vi "LabVIEW2.vi"() -> ()   [LabVIEW 2023]
uses:
  <vilib>/Utility/error.llb/Trim Whitespace One-Sided.vi
panel:
  in  "PNG file path":path=path "/Users/leogallacio/Downloads/N8.png"
  out "concatenated string":string
  out "name":string
  out "Extract path":path
  out "spreadsheet string 2":string
  out "Array 2":string[](array[string])
  out "spreadsheet string":string
  in  "Marker size":i32
  in  "Marker shape":string
  out "Array":u8[][](array[numeric])
  out "appended array":u8[](array[numeric])
  out "B":u8
  out "G":u8
  out "R":u8
  out "size(s)":i32
  out "array":i32[](array[numeric])
  out "before substring":string
  out "after substring":string
  out "Corners":u32(colorbox)
  out "Traces":u32[](array[colorbox])
  out "Color Box":u32(colorbox)
  out "Array with the 6 colors of stdout":i32[](array[numeric])
  out "C:":string
  out "Corners":i32
  out "Color CLUT at index I":u32
  out "CLUT":u32[](array[numeric])
  out "standard error 2":string
  out "standard output 2":string
  out "error out 2":errorcluster
  out "resulting string":string
  out "script.m path":path
  out "return path":path
  out "Traces.txt path":path
  out "name :\nLabVIEW1.vi":string
  out "Traces.txt":string
  out "error out":errorcluster
  out "standard error":string
  out "standard output":string
  out "LabBIEW path :\n/Users/leogallacio/Downloads/LabVIEW":path
  out "Pixmap.bin path":path
  out "profondeur":i32
  out "image":u8[](array[numeric])
  out "largeur":i16
  out "hauteur":i16
  out "PNG picture":picture
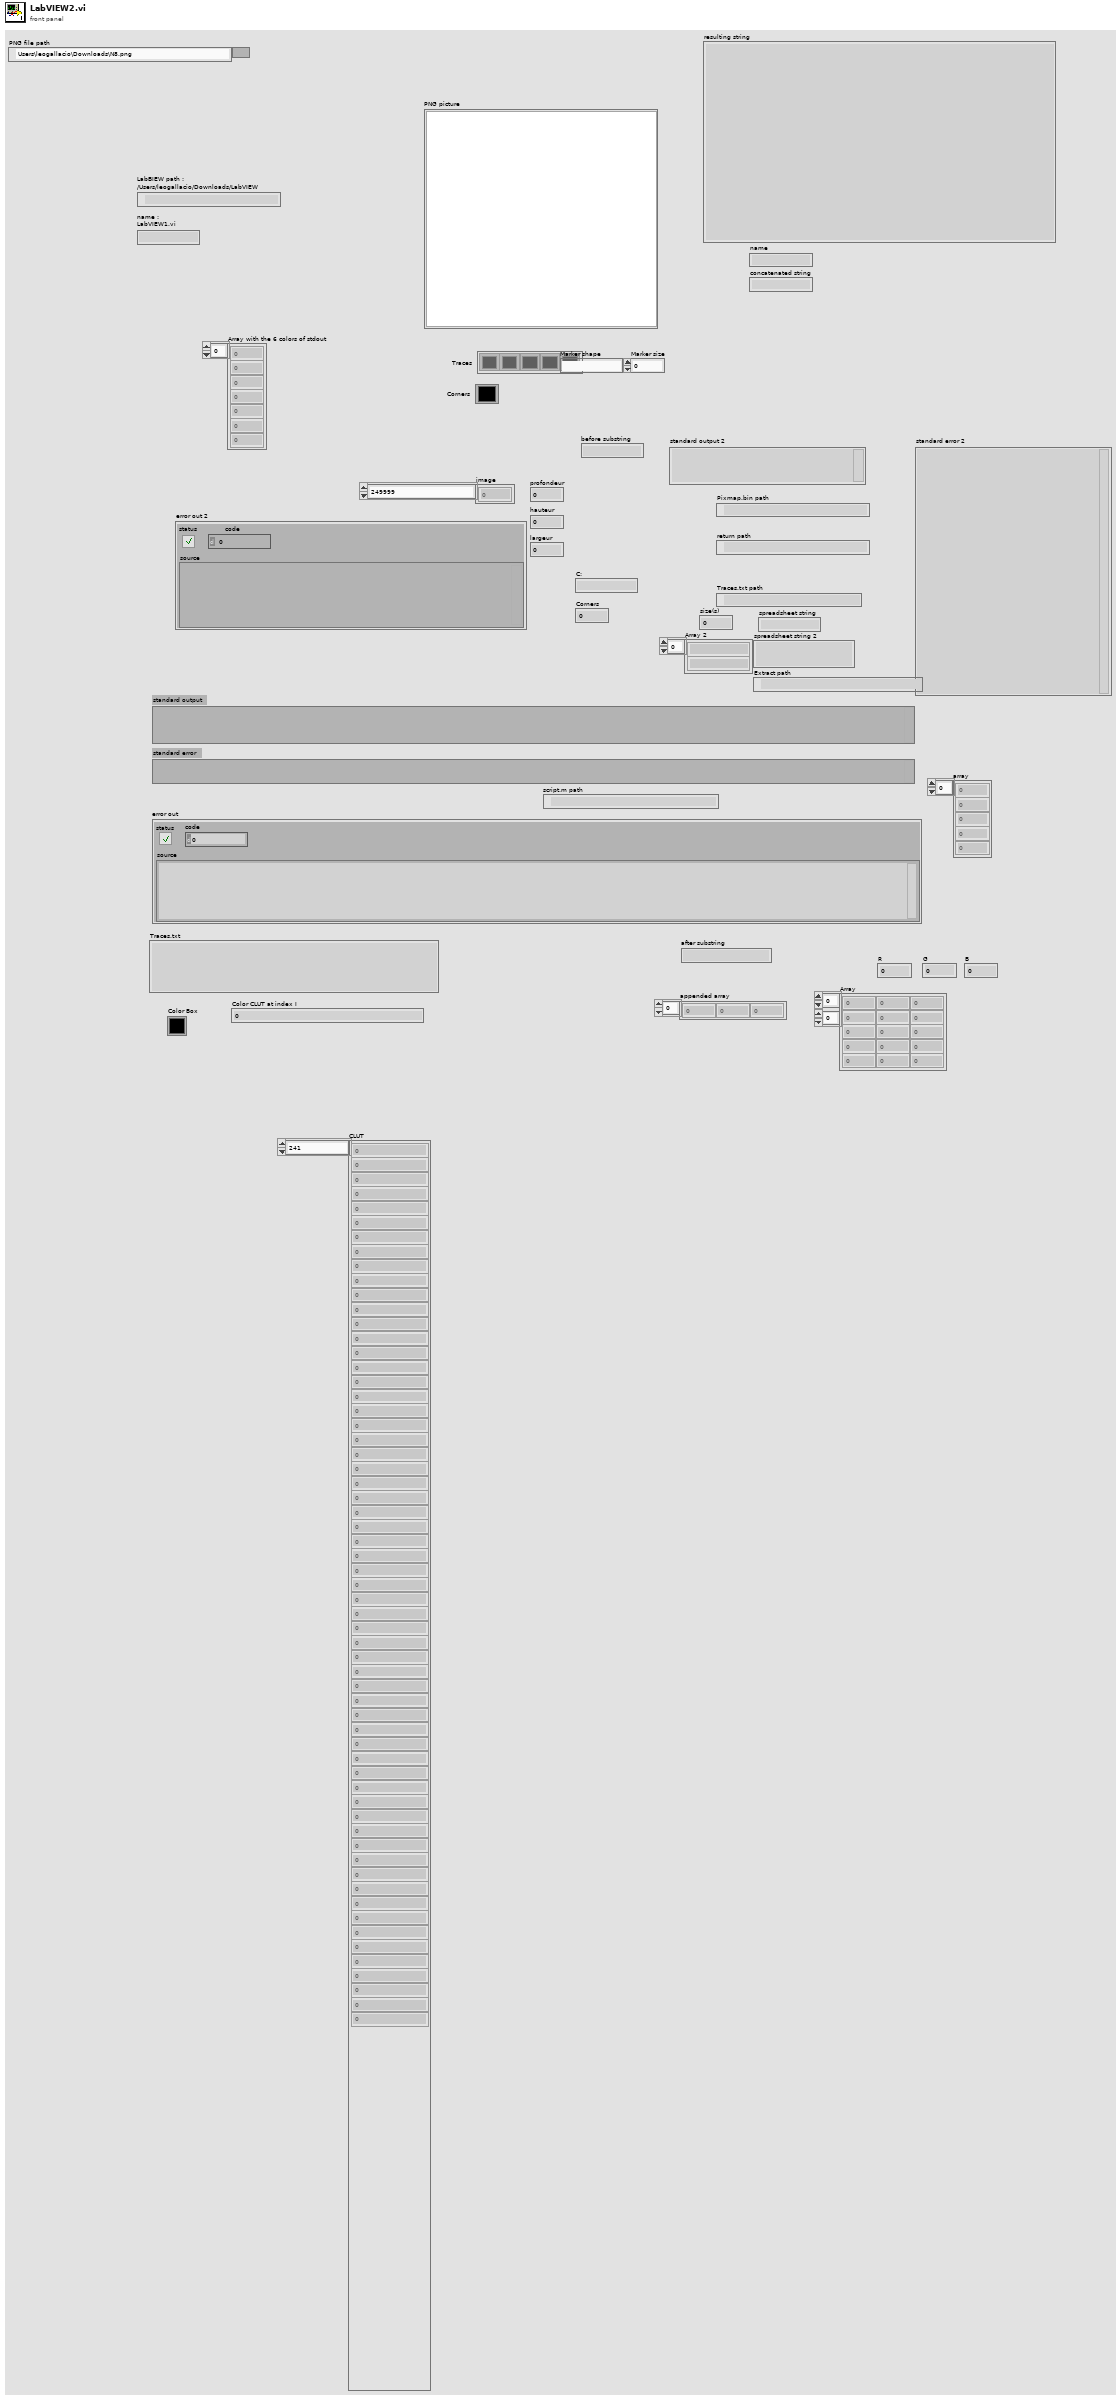
[diagram p1: front panel]
types:
  T1 = enum16{"open", "replace", "create", "open or create", "replace or create", "replace or create with confirmation"}
  T2 = enum16{"big-endian, network order", "native, host order", "little-endian"}
  T3 = typedef "imagedata.ctl" = cluster{"image type":i32, "image depth":i32, "image":u8[], "mask":u8[], "colors":u32[], "Rectangle":cluster{"left":i16, "top":i16, "right":i16, "bottom":i16}}
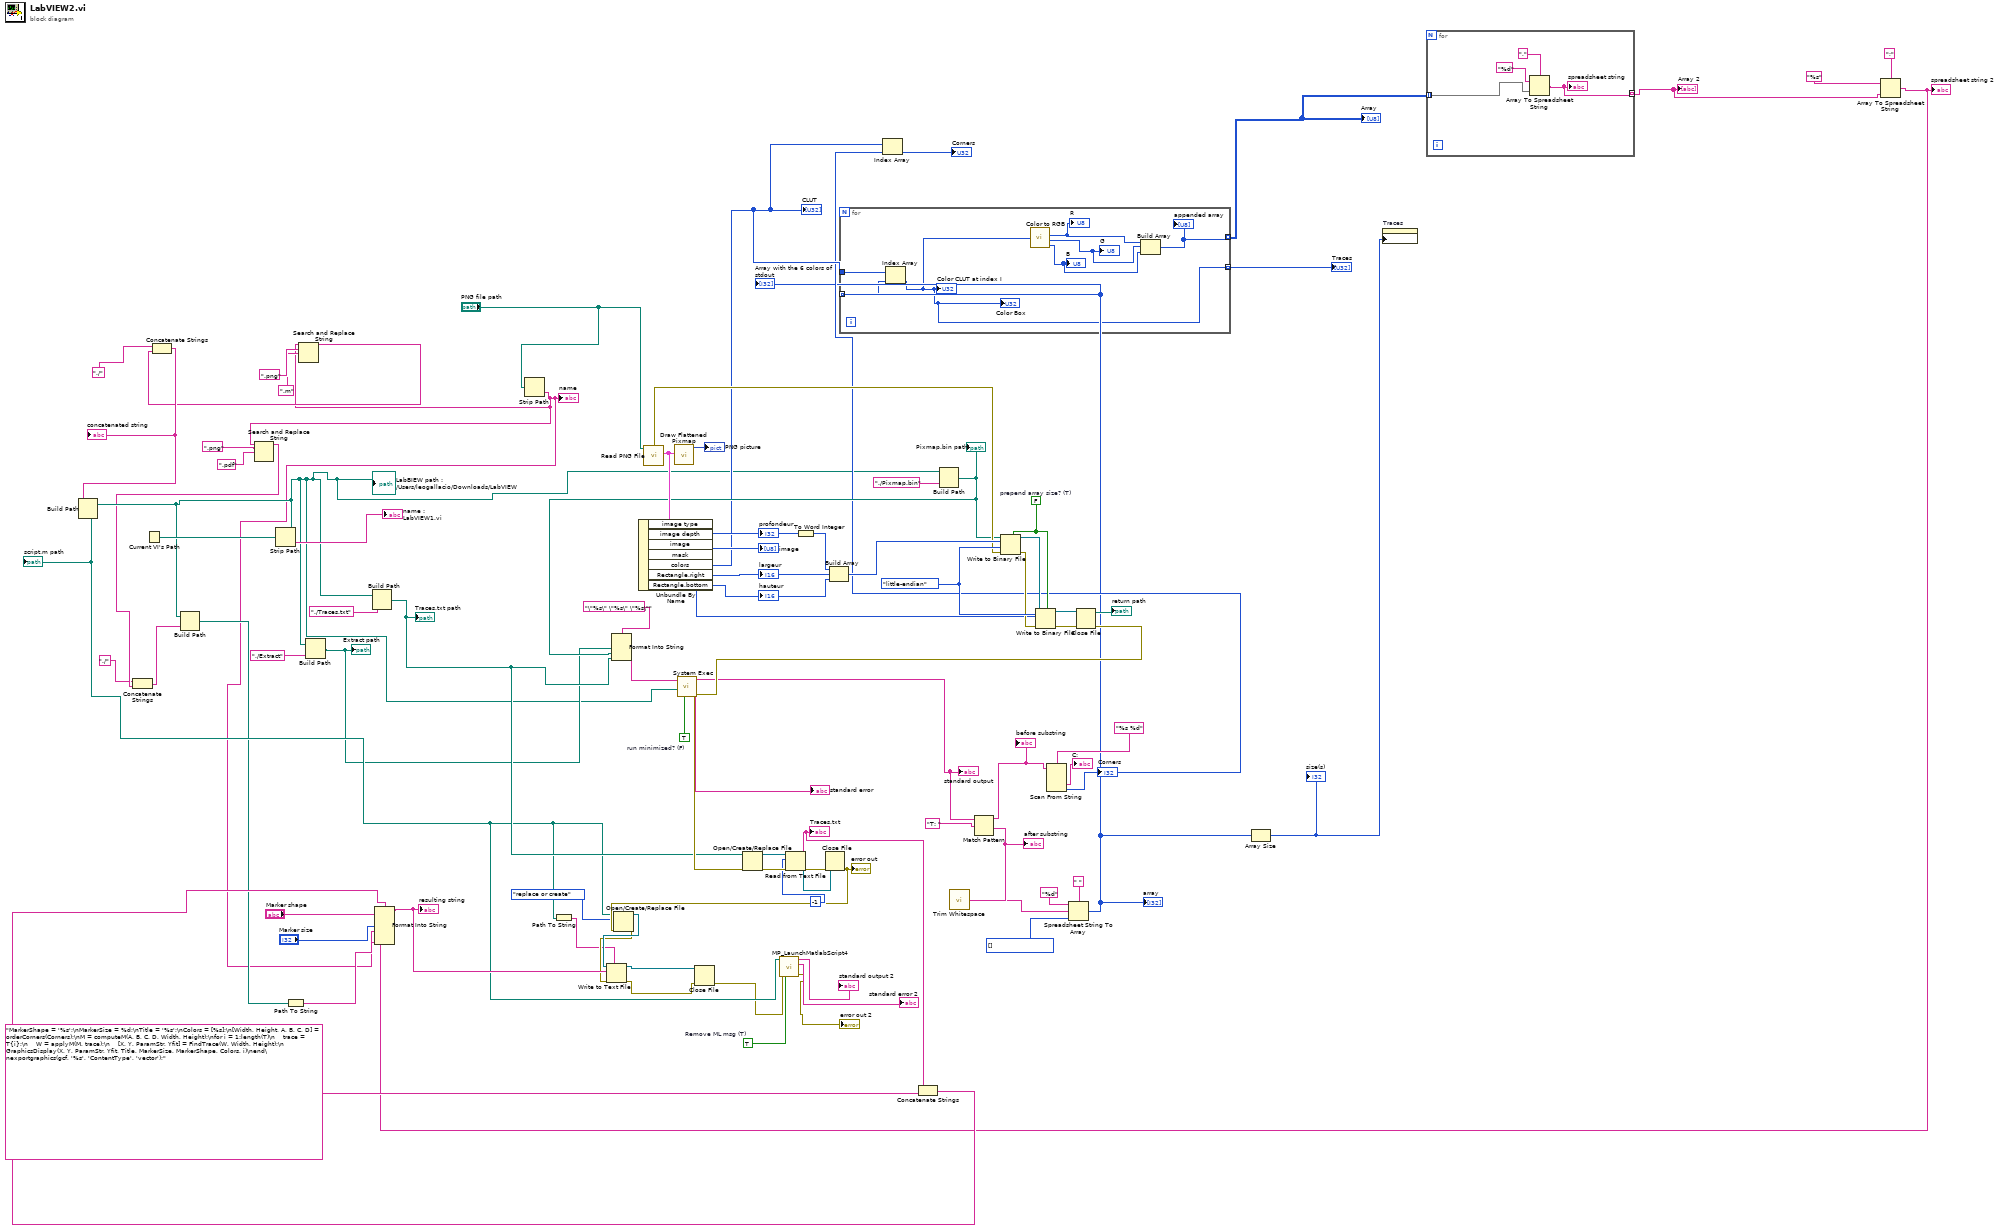
[diagram p0: block diagram]
diagram:
  w19 = TRUE  # Remove ML msg (T)
  w71 = T2."little-endian" ("byte order (0:big-endian, network order)")
  w80 = TRUE  # run minimized? (F)
  w83 = FALSE  # prepend array size? (T)
  n1 = Current VI's Path() -> (path=w73:path)
  n2 = Strip Path(path=w73) -> (stripped path=w8:path, name=→"name :\nLabVIEW1.vi":string)
  "LabBIEW path :\n/Users/leogallacio/Downloads/LabVIEW" <- w8
  n3 = Build Path(base path=w8, name or relative path="./Extract") -> (appended path=w16:path)
  "Extract path" <- w16
  n4 = Build Path(base path=w8, name or relative path="./Traces.txt") -> (appended path=w59:path)
  "Traces.txt path" <- w59
  n5 = Strip Path(path="PNG file path") -> (name=w1:string)  [unwired: 1 out]
  "name" <- w1
  n6 = Search and Replace String(input string=w1, search string=".png", replace string=".pdf" ("replace string (\"\")")) -> (result string=w5:string)  [unwired: 5 in, 3 out]
  n7 = Concatenate Strings("./" ("string"), w5) -> (w3:string)
  n8 = Build Path(base path=w8, name or relative path=w3) -> (appended path=w2:path)
  n9 = Path To String(path=w2) -> (string=w9:string)
  n10 = Search and Replace String(input string=w1, search string=".png", replace string=".m" ("replace string (\"\")")) -> (result string=w10:string)  [unwired: 5 in, 3 out]
  n11 = Concatenate Strings("./" ("string"), w10) -> (w12:string)
  "concatenated string" <- w12
  n12 = Build Path(base path=w8, name or relative path=w12) -> (appended path=w23:path)
  "script.m path" <- w23
  n13 = Path To String(path=w23) -> (string=w52:string)
  n14 = call <vilib>:"Read PNG File.vi"("path to PNG file"="PNG file path") -> ("error out"=w65:errorcluster, "image data"=w74:T3)  [unwired: 8 in, 1 out]
  n15 = Unbundle By Name(w74) -> ("image depth"=w85:i32, "image"=w50:u8[], "colors"=w47:u32[], "Rectangle.right"=w70:i16, "Rectangle.bottom"=w69:i16)  [unwired: 2 out]
  "hauteur" <- w69
  "largeur" <- w70
  "image" <- w50
  "profondeur" <- w85
  "CLUT" <- w47
  n16 = call <vilib>:"Draw Flattened Pixmap.vi"("image data"=w74) -> ("new picture"=→"PNG picture":picture)  [unwired: 8 in]
  n17 = To Word Integer(number=w85) -> (16bit integer=w86:i16)
  n18 = Build Array(w86, w70, w69) -> (w84:i16[])
  n19 = Build Path(base path=w8, name or relative path="./Pixmap.bin") -> (appended path=w63:path)
  "Pixmap.bin path" <- w63
  n20 = Format Into String(format string="\"%s\" \"%s\" \"%s\"", w16, w63, w59) -> (resulting string=w62:string)  [unwired: 2 in, 1 out]
  n21 = Write to Binary File(file (use dialog)=w63, data=w84, error in=w65, 5:w83, 9:w71) -> (refnum out=w87:refnum<file>, error out=w66:errorcluster)  [unwired: 1 in, 1 out]
  n22 = Write to Binary File(file (use dialog)=w87, data=w50, error in=w66, 5:w83, 9:w71) -> (refnum out=w89:refnum<file>, error out=w88:errorcluster)  [unwired: 1 in, 1 out]
  n23 = Close File(refnum=w89, error in=w88) -> (path=→"return path":path, error out=w67:errorcluster)
  n24 = call <vilib>:"System Exec.vi"("run minimized? (F)"=w80, "error in (no error)"=w67, "working directory"=w8, "command line"=w62) -> ("error out"=w72:errorcluster, "standard error"=→"standard error":string, "standard output"=w42:string)  [unwired: 4 in, 1 out]
  "standard output" <- w42
  n25 = Open/Create/Replace File(file path (use dialog)=w59, error in=w72) -> (refnum out=w77:refnum<file>, error out=w79:errorcluster)  [unwired: 4 in, 1 out]
  n26 = Read from Text File(file (use dialog)=w77, count=-1, error in=w79) -> (refnum out=w60:refnum<file>, text=w31:string, error out=w78:errorcluster)  [unwired: 1 in, 1 out]
  "Traces.txt" <- w31
  n27 = Close File(refnum=w60, error in=w78) -> (error out=w56:errorcluster)  [unwired: 1 out]
  "error out" <- w56
  n28 = Open/Create/Replace File(file path (use dialog)=w23, error in=w56, operation (0:open)=T1."replace or create") -> (refnum out=w57:refnum<file>, error out=w55:errorcluster)  [unwired: 3 in, 1 out]
  n29 = Concatenate Strings(w31, "MarkerShape = '%s';\nMarkerSize = %d;\nTitle = '%s';\nColors = [%s];\n[Width, Height, A, B, C, D] = orderCorners(Corners);\nM = computeM(A, B, C, D, Width, Height);\nfor i = 1:length(T)\n    trace = T{i};\n    W = applyM(M, trace);\n    [X, Y, ParamStr, Yfit] = FindTrace(W, Width, Height);\n    GraphicsDisplay(X, Y, ParamStr, Yfit, Title, MarkerSize, MarkerShape, Colors, i)\nend\nexportgraphics(gcf, '%s', 'ContentType', 'vector');" ("initial string")) -> (w29:string)
  n30 = Match Pattern(string=w42, regular expression="T: ") -> (before substring=w41:string, after substring=w38:string)  [unwired: 1 in, 2 out]
  "after substring" <- w38
  "before substring" <- w41
  n31 = call <vilib>:"Trim Whitespace.vi"("string"=w38) -> ("trimmed string"=w37:string)  [unwired: 1 in]
  n32 = Scan From String(format string="%s %d", input string=w41) -> (output 1=→"C:":string, output 2=w46:i32)  [unwired: 4 in, 3 out]
  "Corners" <- w46
  n33 = Index Array(array=w47, index=w46) -> (element=→"Corners":u32)
  n34 = Spreadsheet String To Array(delimiter (Tab)=" ", format string="%d", spreadsheet string=w37, array type (2D Dbl)=i32[] []) -> (array=w35:i32[])
  "Array with the 6 colors of stdout" <- w35
  "array" <- w35
  n35 = for {
    tunnel: w35 -> [w97] mode=indexing
    tunnel: w47 -> [w96]
    tunnel: [w95] -> w36 mode=indexing
    tunnel: [w91] -> w28 mode=indexing
    n36 = Index Array(array=w96, index=w97) -> (element=w95:u32)
    "Color CLUT at index I" <- w95
    "Color Box" <- w95
    n37 = call <vilib>:"Color to RGB.vi"("Color"=w95) -> ("R"=w94:u8, "G"=w93:u8, "B"=w92:u8)  [unwired: 1 out]
    "R" <- w94
    "G" <- w93
    "B" <- w92
    n38 = Build Array(w94, w93, w92) -> (w91:u8[])
    "appended array" <- w91
  }
  "Traces" <- w36
  "Array" <- w28
  n39 = Array Size(array=w35) -> (size(s)=w34:i32)
  "size(s)" <- w34
  n40 = property on="Traces" class="Arr (strict)"("Number of Columns"=w34) -> ()  [unwired: 2 in, 2 out]
  n41 = for {
    tunnel: w28 -> [w101] mode=indexing
    tunnel: [w98] -> w27 mode=indexing
    n42 = Array To Spreadsheet String(delimiter (Tab)=",", array=w101, 3:"%d" ("format string")) -> (spreadsheet string=w98:string)
    "spreadsheet string" <- w98
  }
  "Array 2" <- w27
  n43 = Array To Spreadsheet String(delimiter (Tab)=";", array=w27, 3:"%s" ("format string")) -> (spreadsheet string=w24:string)
  "spreadsheet string 2" <- w24
  n44 = Format Into String(format string=w29, "Marker shape", "Marker size", w1, w24, w9) -> (resulting string=w58:string)  [unwired: 2 in, 1 out]
  "resulting string" <- w58
  n45 = Write to Text File(prompt (Choose or enter file path)=w52, file (use dialog)=w57, text=w58, error in=w55) -> (refnum out=w53:refnum<file>, error out=w54:errorcluster)  [unwired: 1 out]
  n46 = Close File(refnum=w53, error in=w54) -> (error out=w18:errorcluster)  [unwired: 1 out]
  n47 = call "MP_LaunchMatlabScript4.vi"("Remove ML msg (T)"=w19, "error in (no error)"=w18, "matlab script path"=w23) -> ("error out"=→"error out 2":errorcluster, "standard error"=→"standard error 2":string, "standard output"=→"standard output 2":string)  [unwired: 3 in, 3 out]
